vi "GENser Read Instrument Data.vi"(7 "GEN Addr":i16=-1, 8 "error":errorcluster, 10 "Query":string, 11 "VISA":refnum<visa-resource-name>) -> (0 "error out":errorcluster, 1 "Return Count":u32, 2 "Response":string, 3 "VISA out":refnum<visa-resource-name>)   [LabVIEW 2017]
doc: "This VI sends any serial query to the GEN and reads the response message. The Return Count is the number of characters read.\n\nThe Query cannot have a checksum. The checksum is added by the driver. A message terminator is optional. The driver will make the end-of-string to a carriage return.\n\nIf a query error occurs, such as no response message is read because the query is illegal, it is returned in the \"error out\" cluster"
panel:
  # "Read Any Query"
  # "Lambda Genesys \n Serial Port\n  DC Power Supplies"
  # "Includes error checking\n    after query sent\nAdds checksum to qry string"
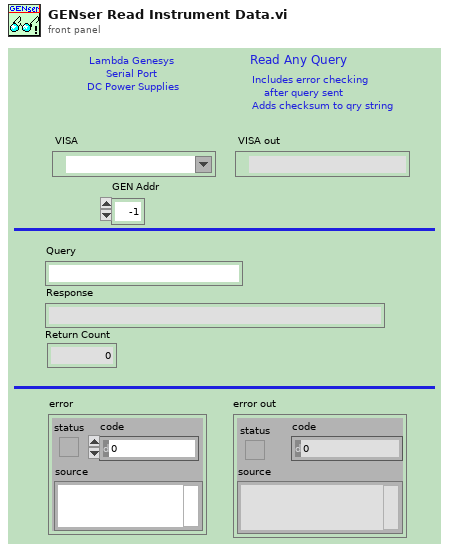
[diagram p1: front panel]
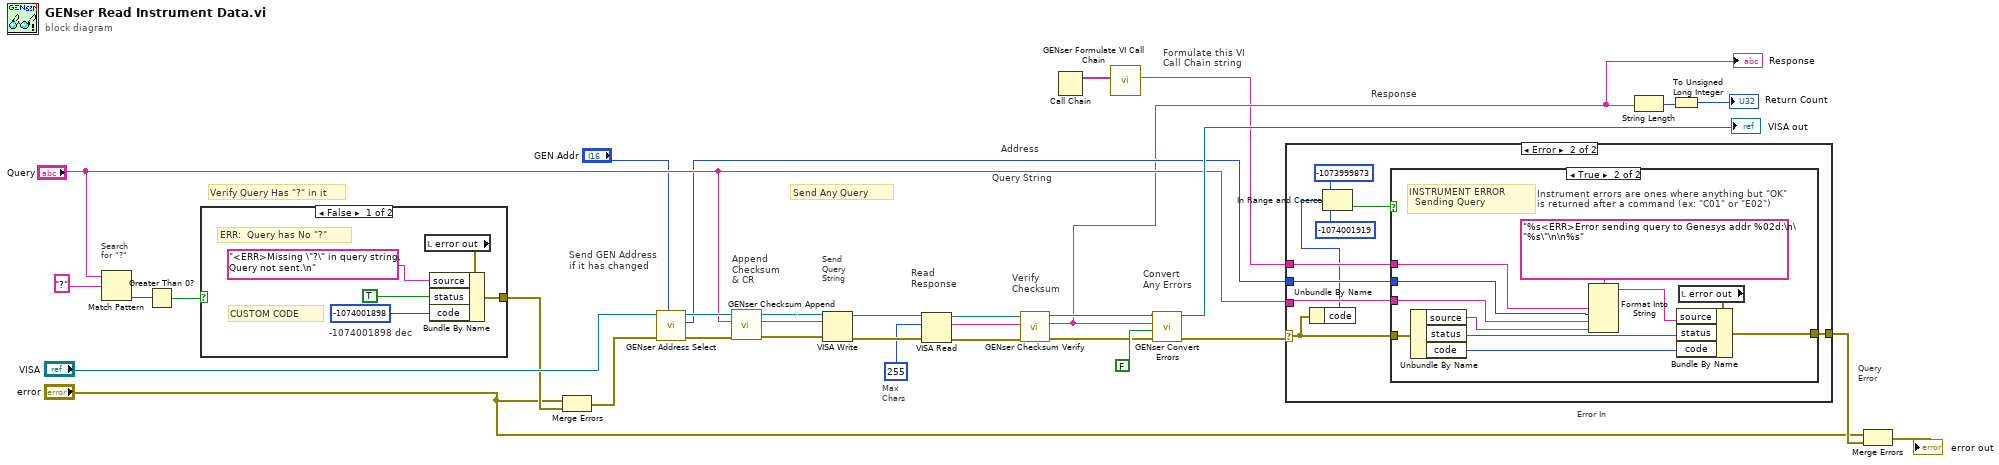
[diagram p0: block diagram]
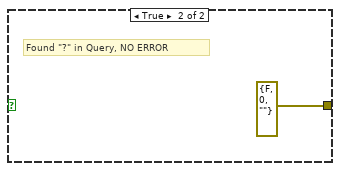
[diagram p4: hidden frame]
diagram:
  # "Address"
  # "Response"
  # "Error In"
  # "Query\nError"
  # "Query String"
  # "Convert\nAny Errors"
  # "Verify\nChecksum"
  # "Append\nChecksum \n& CR"
  # "Send GEN Address\nif it has changed"
  # "Verify Query Has \"?\" in it"
  # "Read\nResponse"
  # "Send\nQuery\nString"
  # "Search\nfor \"?\""
  # "Formulate this VI \nCall Chain string"
  # "Max\nChars"
  # "Send Any Query"
  n1 = Match Pattern(string="Query", regular expression="?") -> (offset past match=w27:i32)  [unwired: 1 in, 3 out]
  n2 = Greater Than 0?(x=w27) -> (x > 0?=w25:bool)
  n3 = case shown="False" w25 {
    tunnel: [w35 errorcluster {"status"=FALSE, "code"=0, "source"=""} ("error out")] -> w24
    frame False {
      # "ERR:  Query has No \"?\""
      # "-1074001898 dec"
      # "CUSTOM CODE"
      n4 = local read "error out"() -> (w38:errorcluster)
      n5 = Bundle By Name(cluster=w38, "source"="<ERR>Missing \"?\" in query string. Query not sent.\n" ("Source"), "status"=TRUE, "code"=-1074001898) -> (w35:errorcluster)
    }
    frame True {
      # "Found \"?\" in Query, NO ERROR"
    }
  }
  n6 = Merge Errors("error", w24) -> (w10:errorcluster)
  n7 = call "GENser Address Select.vi"("GEN Addr"="GEN Addr", "error"=w10, "VISA"="VISA") -> ("error out"=w22:errorcluster, "Last GEN Addr"=w8:i16, "VISA out"=w23:refnum<visa-resource-name>)  [unwired: 6 in]
  n8 = call "GENser Checksum Append.vi"("error"=w22, "Input Cmd"="Query", "VISA"=w23) -> ("error out"=w19:errorcluster, "ChkSum Cmd"=w21:string, "VISA out"=w20:refnum<visa-resource-name>)  [unwired: 6 in]
  n9 = VISA Write(VISA resource name=w20, write buffer=w21, error in (no error)=w19) -> (VISA resource name out=w33:refnum<visa-resource-name>, error out=w32:errorcluster)  [unwired: 1 out]
  n10 = VISA Read(VISA resource name=w33, byte count=u32 255 ("byte count (0)"), error in (no error)=w32) -> (VISA resource name out=w4:refnum<visa-resource-name>, read buffer=w6:string, error out=w3:errorcluster)  [unwired: 1 out]
  n11 = call "GENser Checksum Verify.vi"("error"=w3, "String in"=w6, "VISA"=w4) -> ("error out"=w16:errorcluster, "Trimmed String"=w5:string, "VISA out"=w17:refnum<visa-resource-name>)  [unwired: 6 in]
  "Response" <- w5
  n12 = Call Chain() -> (call chain=w1:string[])
  n13 = call "GENser Formulate VI Call Chain.vi"("Call Chain"=w1) -> ("String Out"=w2:string)  [unwired: 10 in]
  n14 = call "GENser Convert Errors.vi"("error"=w16, "Expect \"OK\" (F)"=FALSE ("Expect \"OK\" (F)"), "String in"=w5, "VISA"=w17) -> ("error out"=w15:errorcluster, "VISA out"=→"VISA out":refnum<visa-resource-name>)  [unwired: 6 in]
  n15 = case shown="Error" w15 {
    selector: w15 -> [w40 w43]
    tunnel: "Query" -> [_ w48]
    tunnel: [w40 w49] -> w12
    tunnel: w2 -> [_ w47]
    tunnel: w8 -> [_ w46]
    frame No Error {
      # "Query Sent Correctly \n  and response Returned"
    }
    frame Error {
      n16 = Unbundle By Name(w43) -> ("code"=w42:i32)
      n17 = In Range and Coerce(upper limit=-1073999873 ("code"), x=w42, lower limit=-1074001919 ("code")) -> (In Range?=w41:bool)  [unwired: 1 out]
      n18 = case shown="True" w41 {
        tunnel: w43 -> [w50 w60]
        tunnel: [w50 w57] -> w49
        tunnel: w48 -> [_ w55]
        tunnel: w47 -> [_ w52]
        tunnel: w46 -> [_ w51]
        frame False {
          # "VISA  ERROR  \n  Sending Command"
          # "For VISA error, do not change error message"
        }
        frame True {
          # "Instrument errors are ones where anything but \"OK\"\nis returned after a command (ex: \"C01\" or \"E02\")"
          # "INSTRUMENT ERROR  \n  Sending Query"
          n19 = Unbundle By Name(w60) -> ("source"=w54:string, "status"=w58:bool, "code"=w59:i32)
          n20 = Format Into String(format string="%s<ERR>Error sending query to Genesys addr %02d:\n\"%s\"\n\n%s" ("Source"), w52, w51, w55, w54) -> (resulting string=w53:string)  [unwired: 2 in, 1 out]
          n21 = local read "error out"() -> (w61:errorcluster)
          n22 = Bundle By Name(cluster=w61, "source"=w53, "status"=w58, "code"=w59) -> (w57:errorcluster)
        }
      }
    }
  }
  n23 = String Length(string=w5) -> (length=w30:i32)
  n24 = To Unsigned Long Integer(number=w30) -> (unsigned 32bit integer=→"Return Count":u32)
  n25 = Merge Errors("error", w12) -> (→"error out":errorcluster)
